vi "Update Listbox.vi"(8 "error in (no error)":errorcluster, 10 "Status Map":map{string, string}(c390), 11 "MulticolumnListbox Reference In":refnum<vi>) -> (0 "error out":errorcluster, 3 "MulticolumnListbox Reference In":refnum<vi>)   [LabVIEW 2020, in "Main.lvclass"]
uses:
  Main.lvclass
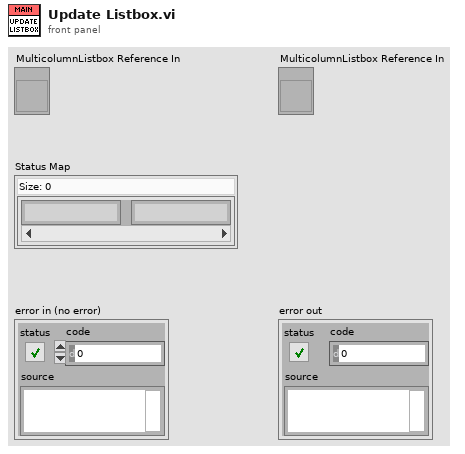
[diagram p1: front panel]
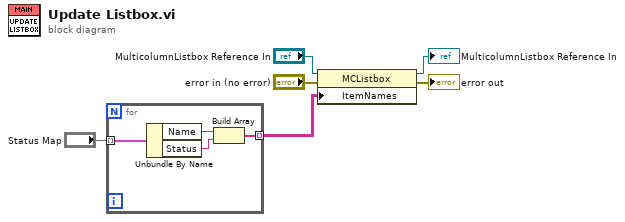
[diagram p0: block diagram]
diagram:
  n1 = for {
    tunnel: [w8] -> w2 mode=indexing
    tunnel: "Status Map" -> [w10] mode=indexing
    n2 = Unbundle By Name(w10) -> ("Name"=w9:string, "Status"=w7:string)
    n3 = Build Array(w9, w7) -> (w8:string[])
  }
  n4 = property class="MCListbox"(reference="MulticolumnListbox Reference In", error in="error in (no error)", "ItemNames"=w2) -> (reference out=→"MulticolumnListbox Reference In":refnum<vi>, error out=→"error out":errorcluster)
